vi "Error - Resource Conflict.vi"   [LabVIEW 2020, in "CTI-Scratchpad.lvlib"]
uses:
  CTI-Scratchpad.lvlib
  CTI/I2C Number.ctl
  CTI/GPIO Number.ctl
  CTI/ADC Number.ctl
  CTI/Session/Session.lvclass
  CTI/CTI.lvlib
  CTI/VisaComms/VisaComms.lvclass
panel:
  # "Configure/run from BD"
types:
  T1 = typedef "CTI.lvlib/ADC Number.ctl" = i8
  T2 = typedef "CTI.lvlib/GPIO Number.ctl" = i8
  T3 = typedef "CTI.lvlib/I2C Number.ctl" = i8
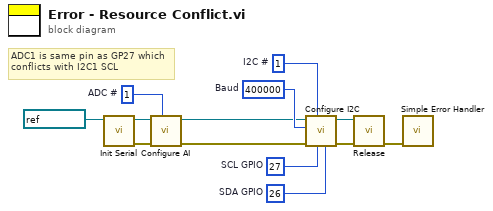
[diagram p0: block diagram]
diagram:
  w1 = T1 1  # ADC #
  w8 = T2 26  # SDA GPIO
  w9 = T2 27  # SCL GPIO
  w10 = T3 1  # I2C #
  w11 = u32 400000  # Baud
  # "ADC1 is same pin as GP27 which conflicts with I2C1 SCL"
  n1 = call "Init Serial.vi"("VISA resource name in"=refnum<visa-resource-name> "COM5" ("Port")) -> ("error out"=w12:errorcluster, "Session"=w3:refnum<class "Session.lvclass">)  [unwired: 8 in, 1 out]
  n2 = call "Configure AI.vi"("ADC #"=w1, "error in (no error)"=w12, "Session in"=w3) -> ("error out"=w4:errorcluster, "Session out"=w2:refnum<class "Session.lvclass">)  [unwired: 7 in]
  n3 = call "Configure I2C.vi"("SDA GPIO"=w8, "SCL GPIO"=w9, "I2C #"=w10, "error in (no error)"=w4, "Baud"=w11, "Session in"=w2) -> ("error out"=w7:errorcluster, "Session out"=w6:refnum<class "Session.lvclass">)  [unwired: 4 in]
  n4 = call-dynamic "Release.vi"("error in (no error)"=w7, "Session in"=w6) -> ("error out"=w5:errorcluster)  [unwired: 9 in]
  n5 = call <vilib>:"Simple Error Handler.vi"("error in (no error)"=w5) -> ()  [unwired: 4 in, 5 out]
